vi "Main.vi"() -> ()   [LabVIEW 2017]
doc: "The myRIO Project template acquires acceleration data from the onboard accelerometer and displays the changes of acceleration values in a waveform chart."
uses:
  <vilib>/Platform/TimedLoop/XDataNode/timing_clust.ctl
  <vilib>/Platform/TimedLoop/XDataNode/nitl_modes.ctl
  <vilib>/Platform/TimedLoop/XDataNode/wakeup.ctl
  <vilib>/myRIO/Common/Instrument Driver Framework/myRIO v1.0/Encoder/typedefs/Encoder Signal Mode.ctl
  <vilib>/myRIO/Instrument Drivers/Onboard IO/Encoder/typedefs/Encoder Reference.ctl
  <vilib>/myRIO/Common/Instrument Driver Framework/Utilities/typedefs/myRIO Generic Hardware Reference.ctl
  <vilib>/myRIO/Common/Instrument Driver Framework/Utilities/typedefs/Hardware Version Enum.ctl
  <vilib>/myRIO/Common/Instrument Driver Framework/Utilities/typedefs/myRIO v1.0 Reference.ctl
  <vilib>/myRIO/Common/Instrument Driver Framework/Utilities/typedefs/Generic FPGA Reference.ctl
  <vilib>/myRIO/Common/Instrument Driver Framework/myRIO v1.0/Encoder/typedefs/Encoder Channels Enum.ctl
  <vilib>/myRIO/Common/Instrument Driver Framework/myRIO v1.0/Encoder/typedefs/Encoder Configuration v1.0.ctl
  <vilib>/userdefined/High Color/nirio_resource_hc.ctl
  <vilib>/myRIO/Common/Instrument Driver Framework/Utilities/vis/Is FPGA Ref Available.vi
  <vilib>/myRIO/Common/Instrument Driver Framework/myRIO v1.0/Encoder/vis/myRIO v1.1 Open Encoder.vi
  <vilib>/myRIO/Instrument Drivers/Onboard IO/Encoder/vis/Read.vi
  <vilib>/myRIO/Common/Instrument Driver Framework/Utilities/vis/Validate Channels.vi
  <vilib>/myRIO/Common/Instrument Driver Framework/myRIO v1.0/Encoder/vis/myRIO v1.0 Reserve Encoder.vi
  <vilib>/myRIO/Common/Instrument Driver Framework/myRIO v1.0/UART/vis/myRIO v1.0 Close UART.vi
  <vilib>/myRIO/Common/Instrument Driver Framework/myRIO v1.0/Encoder/vis/myRIO v1.0 Build MUX Configuration Encoder.vi
  <vilib>/myRIO/Common/Instrument Driver Framework/myRIO v1.0/Resource Manager/vis/myRIO v1.0 Reserve Channel List.vi
  <vilib>/myRIO/Common/Instrument Driver Framework/myRIO v1.0/Resource Manager/vis/myRIO v1.0 Create Configuration List.vi
  <vilib>/myRIO/Common/Instrument Driver Framework/myRIO v1.0/Resource Manager/vis/myRIO v1.0 Reserve Channel.vi
  <vilib>/myRIO/Common/Instrument Driver Framework/myRIO v1.0/Resource Manager/vis/myRIO v1.0 Unreserve Channel.vi
  <vilib>/myRIO/Common/Instrument Driver Framework/myRIO v1.0/Resource Manager/vis/myRIO v1.0 Build Mutex Name.vi
  Inputs.vi
  Outputs.vi
  <vilib>/addons/control/pid/pid.llb/PID (DBL).vi
  <vilib>/Utility/VariantDataType/GetNumericInfo.vi
  <vilib>/Utility/error.llb/Error Cluster From Error Code.vi
  <vilib>/myRIO/Common/Instrument Driver Framework/myRIO v1.0/myRIO v1.1 Open.vi
  <vilib>/myRIO/Common/Instrument Driver Framework/Utilities/vis/IO Manager.vi
  <vilib>/myRIO/Common/Instrument Driver Framework/Utilities/vis/Configuration Manager.vi
  <vilib>/myRIO/Common/Instrument Driver Framework/myRIO v1.0/Resource Manager/vis/myRIO v1.0 Configure IO.vi
  <vilib>/myRIO/Common/Instrument Driver Framework/myRIO v1.0/myRIO v1.0 Close.vi
  <vilib>/myRIO/Common/Instrument Driver Framework/myRIO v1.0/Encoder/vis/myRIO v1.0 Configure Encoder.vi
  <vilib>/myRIO/Common/Instrument Driver Framework/myRIO v1.0/Encoder/vis/myRIO v1.0 Read Encoder.vi
  <vilib>/myRIO/Common/Instrument Driver Framework/Utilities/vis/FPGA Ref Manager.vi
  <vilib>/myRIO/Common/Instrument Driver Framework/myRIO v1.0/myRIO v1.0 Reset FPGA.vi
  <vilib>/myRIO/Common/Instrument Driver Framework/myRIO v1.0/IRQ/vis/myRIO v1.0 IRQ Info FGV.vi
  <vilib>/myRIO/Common/Instrument Driver Framework/myRIO v1.0/IRQ/vis/myRIO v1.0 Timer IRQ Info FGV.vi
  <vilib>/myRIO/Common/Instrument Driver Framework/myRIO v1.0/IRQ/vis/myRIO v1.0 ISR Agent.vi
  <vilib>/platform/TimedLoop/XDataNode/XDataNode.xnode
  <vilib>/myRIO/Express VI/Onboard IO/Encoder/Encoder Express VI.xnode
  <vilib>/myRIO/Instrument Drivers/Onboard IO/Encoder/vis/myRIO Encoder Open.xnode
  <vilib>/myRIO/Common/Instrument Driver Framework/myRIO v1.0/Encoder/typedefs/Encoder Count Direction Enum.ctl
  <vilib>/myRIO/Instrument Drivers/Utilities/Utilities.lvlib
  <vilib>/myRIO/Instrument Drivers/Onboard IO/Encoder/Encoder.lvlib
  <vilib>/Platform/TimedLoop/XDataNode/XDNodeRunTimeDep.lvlib
  <vilib>/addons/control/pid/NI_PID_pid.lvlib
panel:
  out "Waveform Chart":dbl(graph)
  in  "Acc":dbl format="%.2f"
  in  "Speed":dbl format="%.2f"
  in  "Stop":bool
  out "Boolean 2":bool=TRUE
  in  "setpoint":dbl format="%.2f"
  in  "PID gains":T1={"proportional gain (Kc)"=1.0, "integral time (Ti, min)"=0.01, "derivative time (Td, min)"=0.0} {"derivative time (Td, min)" format="%.3f"; "integral time (Ti, min)" format="%.3f"; "proportional gain (Kc)" format="%.3f"}
  out "X":dbl
  out "error out":errorcluster
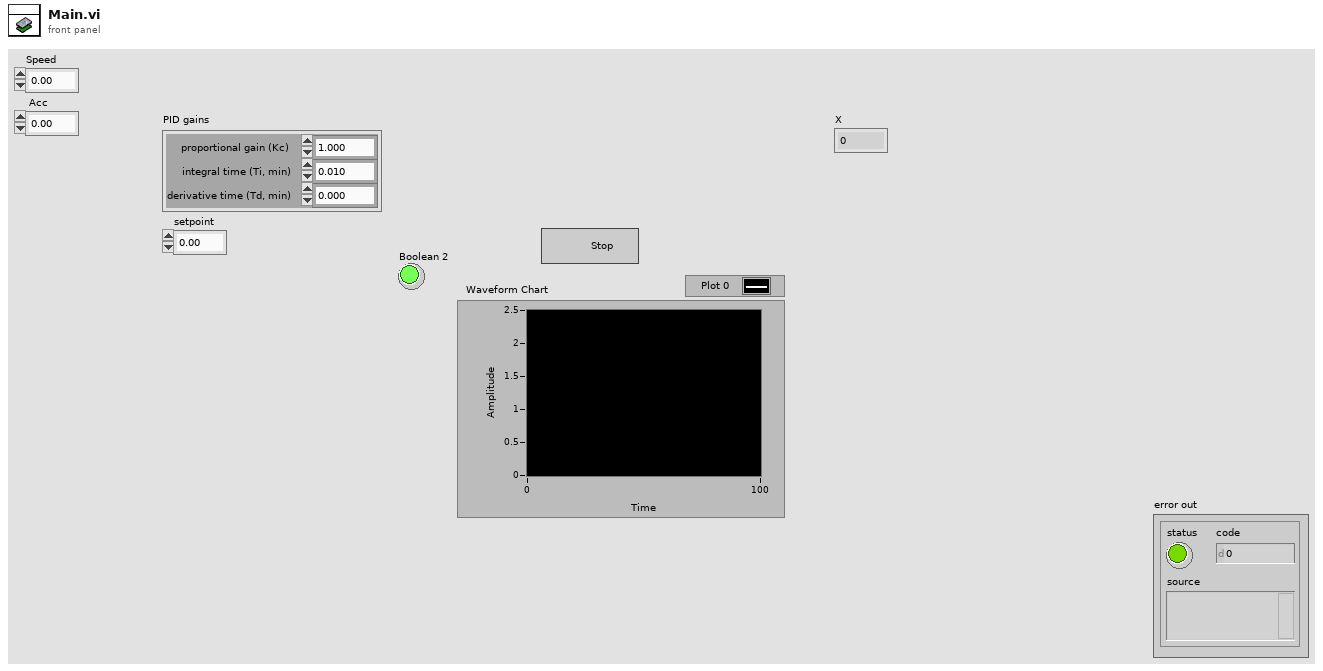
[diagram p1: front panel]
types:
  T1 = cluster{"proportional gain (Kc)":dbl, "integral time (Ti, min)":dbl, "derivative time (Td, min)":dbl}
  T2 = typedef "XDNodeRunTimeDep.lvlib/timing_clust.ctl" = cluster{"Expected End [f-1]":u64, "Actual End [f-1]":u64, "Finished Late? [f-1]":bool, "Expected End [i-1]":u64, "Actual End [i-1]":u64, "Finished Late? [i-1]":bool, "Expected Start [i]":u64, "Actual Start [i]":u64, "Expected Start [f]":u64, "Actual Start [f]":u64, "Source Name":string, "Structure Name":string, "Period":i64, "Deadline":i64, "Offset":i64, "Start":i64, "Priority":i32, "Timeout":i32, "Mode":T3, "Wakeup Reason":T4, "Error":errorcluster, "Source Type":string, "Secondary Source Type":string, "Global End Time":u64, "Global Start Time":u64, "Frame Duration":u64, "Iteration Duration":u64, "Assigned CPU":i32, "I/O Scan Engine Mode":u32}
  T3 = typedef "XDNodeRunTimeDep.lvlib/nitl_modes.ctl" = enum32{"No Change", "Process missed periods, maintain original phase", "Discard missed periods, maintain original phase", "Process missed periods, ignore original phase", "Discard missed periods, ignore original phase"}
  T4 = typedef "XDNodeRunTimeDep.lvlib/wakeup.ctl" = enum32{"Normal", "Aborted", "Asynchronous wakeup", "Timing source error", "Timed loop error", "Timeout"}
  T5 = typedef "Encoder.lvlib/Encoder Reference.ctl" = cluster{"myRIO Reference":T6, "Encoder Channels Enum":T10}
  T6 = typedef "myRIO Generic Hardware Reference.ctl" = cluster{"myRIO Model":T7, "myRIO Hardware Reference":T8}
  T7 = typedef "Hardware Version Enum.ctl" = enum16{"Unknown", "myRIO-1900", "myRIO-1950", "roboRIO", "NI ELVIS RIO CM"}
  T8 = typedef "myRIO v1.0 Reference.ctl" = cluster{"Generic FPGA Reference":T9, "Allow multiple opens":bool}
  T9 = typedef "Generic FPGA Reference.ctl" = refnum<k20>
  T10 = typedef "Encoder Channels Enum.ctl" = enum16{"Not Connected", "C/ENC0", "C/ENC1", "A/ENC", "B/ENC", "DIO/ENC0", "DIO/ENC1", "DIO/ENC2", "DIO/ENC3", "DIO/ENC4"}
  T11 = typedef "Encoder Signal Mode.ctl" = enum16{"Quadrature phase signal", "Step and direction signal"}
  T12 = typedef "nirio_resource_hc.ctl" = tag
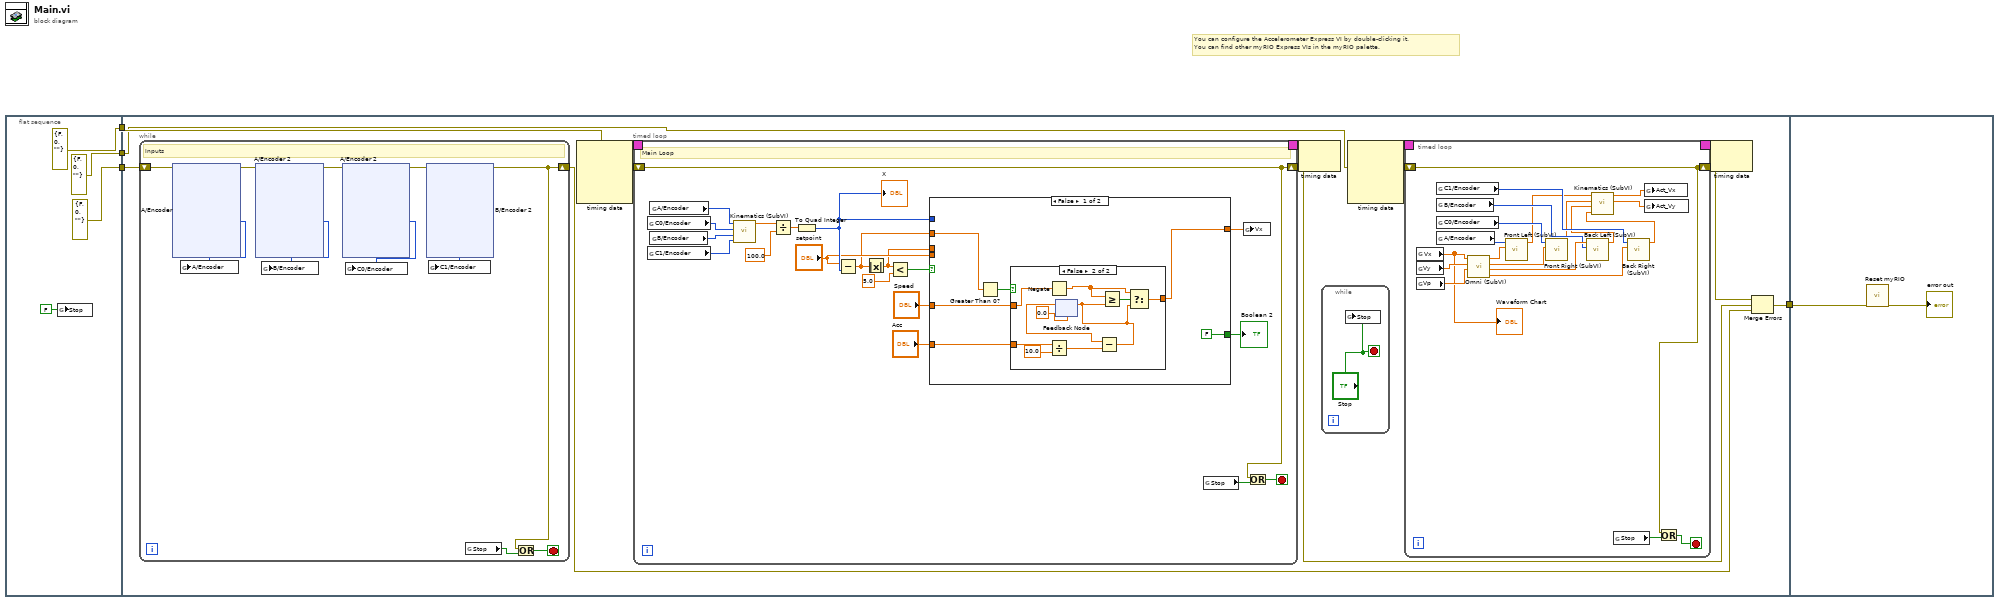
[diagram p0: block diagram]
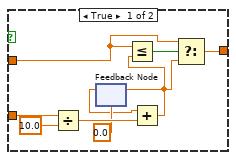
[diagram p2: hidden frame]
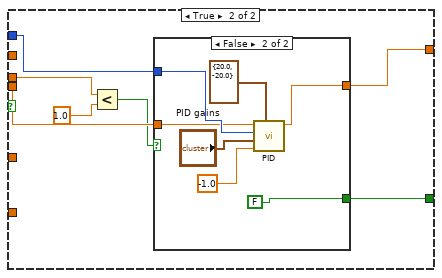
[diagram p3: hidden frame]
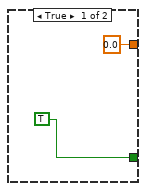
[diagram p4: hidden frame]
diagram:
  # "You can configure the Accelerometer Express VI by double-clicking it.\nYou can find other myRIO Express VIs in the myRIO palette."
  n1 = flat-sequence {
    tunnel: [errorcluster {"status"=FALSE, "code"=0, "source"=""} ("error in (no error)")] -> w4
    tunnel: [errorcluster {"status"=FALSE, "code"=0, "source"=""} ("error in (no error)")] -> w2
    tunnel: [errorcluster {"status"=FALSE, "code"=0, "source"=""} ("error in (no error)")] -> w1
    tunnel: w4 -> [w19]
    tunnel: [w13] -> w3
    tunnel: w2 -> [w10]
    tunnel: w1 -> [w9]
    tunnel: w3 -> [w305]
    frame #0 {
      # "Initialize"
      n2 = global write "Inputs.vi" "Stop"(FALSE ("Stop")) -> ()
    }
    frame #1 {
      n3 = while {
        shift-right: [w110] -> w11
        shift-left: w19 -> [w117]
        stop <- w111 stop-if-true
        # "Inputs"
        n4 = xnode "A/Encoder"("error in (no error)"=w117) -> ("Counter Value"=w120:i32, "error out"=w118:errorcluster)  [unwired: 1 in, 2 out]
        n5 = global write "Inputs.vi" "A/Encoder"(w120) -> ()
        n6 = xnode "A/Encoder 2"("error in (no error)"=w118) -> ("Counter Value"=w119:i32, "error out"=w114:errorcluster)  [unwired: 1 in, 2 out]
        n7 = global write "Inputs.vi" "B/Encoder"(w119) -> ()
        n8 = xnode "A/Encoder 2"("error in (no error)"=w114) -> ("Counter Value"=w116:i32, "error out"=w113:errorcluster)  [unwired: 1 in, 2 out]
        n9 = global write "Inputs.vi" "C0/Encoder"(w116) -> ()
        n10 = xnode "B/Encoder 2"("error in (no error)"=w113) -> ("Counter Value"=w115:i32, "error out"=w110:errorcluster)  [unwired: 1 in, 2 out]
        n11 = global write "Inputs.vi" "C1/Encoder"(w115) -> ()
        n12 = global read "Inputs.vi" "Stop"() -> (w112:bool)
        n13 = Or(x=w110, y=w112) -> (x .or. y?=w111:bool)
      }
      n14 = node-c288() -> (w16:T2)  [unwired: 4 in]
      n15 = timed-loop {
        shift-right: [w28] -> w12
        shift-left: w10 -> [w28]
        timing: w16 -> [_]
        timing-out: [_] -> w15
        stop <- w39 stop-if-true
        # "Main Loop"
        n16 = global read "Inputs.vi" "C0/Encoder"() -> (w36:i32)
        n17 = global read "Inputs.vi" "C1/Encoder"() -> (w34:i32)
        n18 = global read "Inputs.vi" "A/Encoder"() -> (w37:i32)
        n19 = global read "Inputs.vi" "B/Encoder"() -> (w35:i32)
        n20 = call "Kinematics (SubVI).vi"("Forward Left"=w37, "Forward Right"=w36, "Back Left"=w35, "Back Right"=w34) -> ("X"=w33:dbl)  [unwired: 5 in, 1 out]
        n21 = Divide(x=w33, y=100.0) -> (x/y=w31:dbl)
        n22 = To Quad Integer(1:w31) -> (0:w23:i64)
        "X" <- w23
        n23 = Subtract(x="setpoint", y=w23) -> (x-y=w21:dbl)
        n24 = Absolute Value(x=w21) -> (abs(x)=w20:dbl)
        n25 = Less?(x=w20, y=5.0) -> (x < y?=w29:bool)
        n26 = case shown="False" w29 {
          tunnel: w23 -> [_ w68]
          tunnel: [w41 w71] -> w27
          tunnel: "setpoint" -> [_ w69]
          tunnel: "Speed" -> [w45 _]
          tunnel: "Acc" -> [w44 _]
          tunnel: w21 -> [w43 _]
          tunnel: [FALSE ("Boolean") w66] -> w24
          tunnel: w20 -> [_ w65]
          frame False {
            n27 = Greater Than 0?(x=w43) -> (x > 0?=w42:bool)
            n28 = case shown="False" w42 {
              tunnel: w45 -> [w50 w55]
              tunnel: w44 -> [w53 w63]
              tunnel: [w49 w60] -> w41
              frame True {
                n29 = Divide(x=w53, y=10.0) -> (x/y=w51:dbl)
                n30 = feedback #1(0.0) -> (w47:dbl)
                n31 = Add(x=w47, y=w51) -> (x+y=w46:dbl)
                n32 = feedback-in #1(w46) -> ()
                n33 = Less Or Equal?(x=w50, y=w46) -> (x <= y?=w54:bool)
                n34 = Select(t=w50, s=w54, f=w46) -> (s? t:f=w49:dbl)
              }
              frame False {
                n35 = Negate(x=w55) -> (-x=w56:dbl)
                n36 = Divide(x=w63, y=10.0) -> (x/y=w61:dbl)
                n37 = feedback #2(0.0) -> (w59:dbl)
                n38 = Subtract(x=w59, y=w61) -> (x-y=w58:dbl)
                n39 = feedback-in #2(w58) -> ()
                n40 = Greater Or Equal?(x=w56, y=w58) -> (x >= y?=w64:bool)
                n41 = Select(t=w56, s=w64, f=w58) -> (s? t:f=w60:dbl)
              }
            }
          }
          frame True {
            n42 = Less?(x=w65, y=1.0) -> (x < y?=w67:bool)
            n43 = case shown="False" w67 {
              tunnel: w68 -> [_ w80]
              tunnel: [0.0 ("output") w79] -> w71
              tunnel: w69 -> [_ w78]
              tunnel: [TRUE ("Boolean") FALSE ("Boolean")] -> w66
              frame True {
              }
              frame False {
                n44 = call-poly <vilib>:"PID.vi"("output range"=cluster{"output high":dbl, "output low":dbl} {"output high"=20.0, "output low"=-20.0}, "dt (s)"=-1.0, "PID gains"="PID gains", "process variable"=w80, "setpoint"=w78) -> ("output"=w79:dbl)  [unwired: 5 in, 1 out]
              }
            }
          }
        }
        "Boolean 2" <- w24
        n45 = global read "Inputs.vi" "Stop"() -> (w38:bool)
        n46 = global write "Outputs.vi" "Vx"(w27) -> ()
        n47 = Or(x=w28, y=w38) -> (x .or. y?=w39:bool)
      }
      n48 = node-c288(w15) -> ()  [unwired: 1 out]
      n49 = while {
        stop <- "Stop" stop-if-true
        n50 = global write "Inputs.vi" "Stop"("Stop") -> ()
      }
      n51 = node-c288() -> (w18:T2)  [unwired: 4 in]
      n52 = timed-loop {
        timing: w18 -> [_]
        timing-out: [_] -> w17
        shift-right: [w86] -> w14
        shift-left: w9 -> [w86]
        stop <- w87 stop-if-true
        n53 = global read "Outputs.vi" "Vy"() -> (w92:dbl)
        n54 = global read "Outputs.vi" "Vp"() -> (w91:dbl)
        n55 = global read "Outputs.vi" "Vx"() -> (w85:dbl)
        "Waveform Chart" <- w85
        n56 = global read "Inputs.vi" "C1/Encoder"() -> (w97:i32)
        n57 = global read "Inputs.vi" "B/Encoder"() -> (w99:i32)
        n58 = global read "Inputs.vi" "C0/Encoder"() -> (w98:i32)
        n59 = global read "Inputs.vi" "A/Encoder"() -> (w104:i32)
        n60 = call "Omni (SubVI).vi"("Vp"=w91, "Vy"=w92, "Vx"=w85) -> ("Back_Right"=w100:dbl, "Back_Left"=w101:dbl, "Front_Right"=w102:dbl, "Front_Left"=w103:dbl)  [unwired: 4 in]
        n61 = call "Front Left (SubVI).vi"("setpoint"=w103, "Counter Value"=w104) -> ("speed"=w93:dbl)  [unwired: 8 in, 1 out]
        n62 = call "Front Right (SubVI).vi"("setpoint"=w102, "Counter Value"=w98) -> ("speed"=w94:dbl)  [unwired: 8 in, 1 out]
        n63 = call "Back Left (SubVI).vi"("Counter input"=w99, "setpoint"=w101) -> ("speed"=w95:dbl)  [unwired: 8 in, 1 out]
        n64 = global read "Inputs.vi" "Stop"() -> (w88:bool)
        n65 = call "Back Right (SubVI).vi"("setpoint"=w100, "Counter Value"=w97) -> ("speed"=w96:dbl)  [unwired: 8 in, 1 out]
        n66 = call "Kinematics (SubVI).vi"("Forward Left"=w93, "Forward Right"=w94, "Back Left"=w95, "Back Right"=w96) -> ("X"=w89:dbl, "Y"=w90:dbl)  [unwired: 5 in]
        n67 = global write "Inputs.vi" "Act_Vx"(w89) -> ()
        n68 = global write "Inputs.vi" "Act_Vy"(w90) -> ()
        n69 = Or(x=w86, y=w88) -> (x .or. y?=w87:bool)
      }
      n70 = node-c288(w17) -> ()  [unwired: 1 out]
      n71 = Merge Errors(w14, w12, w11) -> (w13:errorcluster)
    }
    frame #2 {
      # "Close"
      n72 = call <vilib>:"Reset myRIO.vi"("error in (no error)"=w305) -> ("error out"=→"error out":errorcluster)  [unwired: 10 in]
    }
  }
